vi "salRegSubEventsCMDsDL.vi"(8 "error in (no error)":errorcluster, 11 "MiddlewareSALThisComponent in":refnum<class "MiddlewareSALThisComponent.lvclass">) -> (0 "error out":errorcluster, 2 "Event Registration Refnum":refnum<event-registration>, 3 "MiddlewareSALThisComponent out":refnum<class "MiddlewareSALThisComponent.lvclass">)   [LabVIEW 2016, in "MiddlewareSALThisComponent.lvclass"]
uses:
  MiddlewareSALThisComponent.lvclass
  <vilib>/Utility/error.llb/DialogType.ctl
  ProgrammaticInitialization/ProgrammaticInitialization.lvclass
  ts_sallv_sedspectrometer/SALLV_calibrationSpectrometer.lvlib
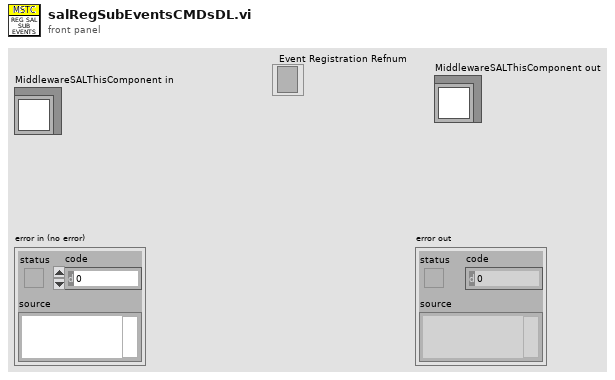
[diagram p1: front panel]
types:
  T1 = typedef "DialogType.ctl" = u16
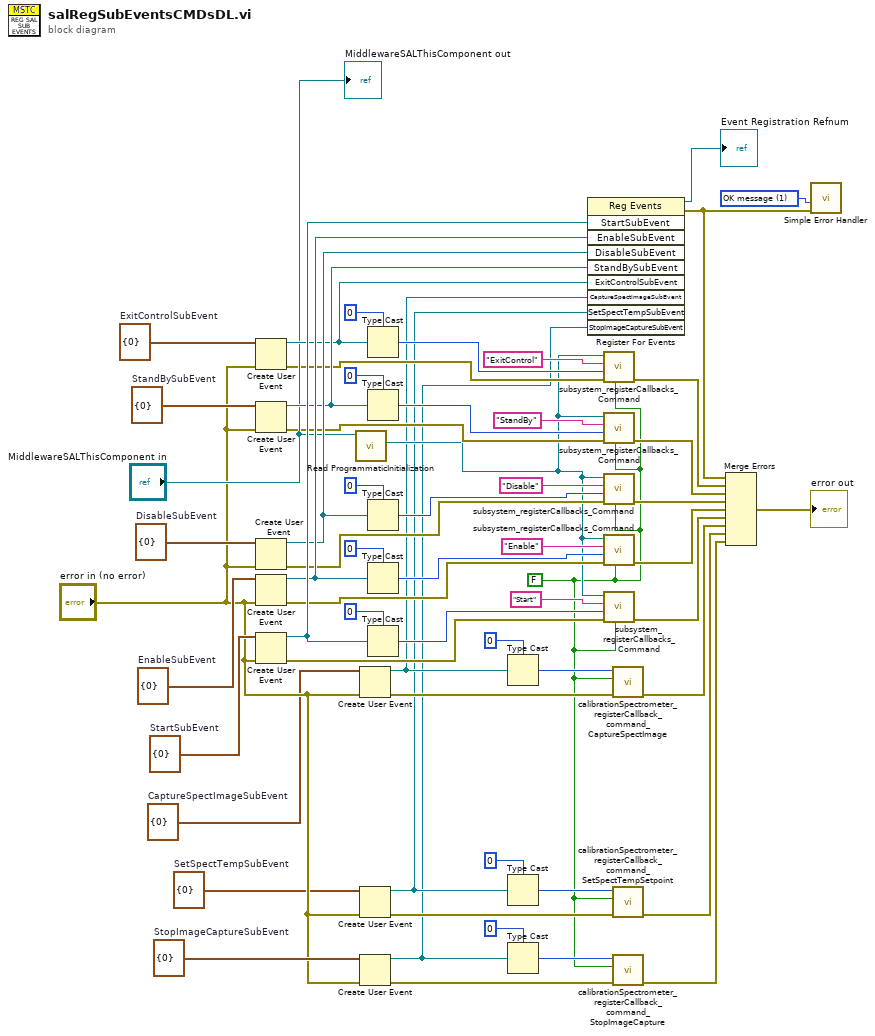
[diagram p0: block diagram]
diagram:
  w22 = cluster{"Data":i32} {"Data"=0}  # StopImageCaptureSubEvent
  w16 = cluster{"Data":i32} {"Data"=0}  # CaptureSpectImageSubEvent
  w20 = cluster{"Data":i32} {"Data"=0}  # SetSpectTempSubEvent
  w47 = cluster{"Data":i32} {"Data"=0}  # ExitControlSubEvent
  w49 = cluster{"Data":i32} {"Data"=0}  # StandBySubEvent
  w54 = cluster{"Data":i32} {"Data"=0}  # DisableSubEvent
  w57 = cluster{"Data":i32} {"Data"=0}  # EnableSubEvent
  w60 = cluster{"Data":i32} {"Data"=0}  # StartSubEvent
  w61 = T1 1 items=["no dialog", "OK message", "continue or stop message", "OK message + warnings", "continue/stop + warnings"] ("type of dialog (OK msg:1)")
  w4 = FALSE ("skipOld")
  n1 = Create User Event(user event datatype=w47, error in="error in (no error)") -> (user event=w46:refnum<user-event>, error out=w33:errorcluster)
  n2 = Create User Event(user event datatype=w49, error in="error in (no error)") -> (user event=w50:refnum<user-event>, error out=w32:errorcluster)
  n3 = Create User Event(user event datatype=w54, error in="error in (no error)") -> (user event=w52:refnum<user-event>, error out=w31:errorcluster)
  n4 = Create User Event(user event datatype=w57, error in="error in (no error)") -> (user event=w55:refnum<user-event>, error out=w28:errorcluster)
  n5 = Create User Event(user event datatype=w60, error in="error in (no error)") -> (user event=w58:refnum<user-event>, error out=w25:errorcluster)
  n6 = call-dynamic "Read ProgrammaticInitialization.vi"("MiddlewareSALThisComponent in"="MiddlewareSALThisComponent in") -> ("ProgrammaticInitialization"=w15:refnum<class "ProgrammaticInitialization.lvclass">)  [unwired: 8 in, 2 out]
  n7 = Create User Event(user event datatype=w16, error in="error in (no error)") -> (user event=w3:refnum<user-event>, error out=w12:errorcluster)
  n8 = Create User Event(user event datatype=w20, error in="error in (no error)") -> (user event=w2:refnum<user-event>, error out=w8:errorcluster)
  n9 = Create User Event(user event datatype=w22, error in="error in (no error)") -> (user event=w1:refnum<user-event>, error out=w7:errorcluster)
  n10 = Type Cast(type=0, x=w46) -> (*(type *) &x=w43:i32)
  n11 = Type Cast(type=0, x=w50) -> (*(type *) &x=w38:i32)
  n12 = Type Cast(type=0, x=w52) -> (*(type *) &x=w35:i32)
  n13 = Type Cast(type=0, x=w55) -> (*(type *) &x=w30:i32)
  n14 = Type Cast(type=0, x=w58) -> (*(type *) &x=w24:i32)
  n15 = Type Cast(type=0, x=w3) -> (*(type *) &x=w13:i32)
  n16 = Type Cast(type=0, x=w2) -> (*(type *) &x=w9:i32)
  n17 = Type Cast(type=0, x=w1) -> (*(type *) &x=w5:i32)
  n18 = register-events(w58, w55, w52, w50, w46, w3, w2, w1) -> (reference out=→"Event Registration Refnum":refnum<event-registration>, error out=w45:errorcluster)  [unwired: 2 in]
  n19 = call "subsystem_registerCallbacks_Command.vi"("skipOld"=w4, "error in (no error)"=w33, "handle"=w43, "topic"="ExitControl", "ProgrammaticInitialization in"=w15) -> ("error out"=w42:errorcluster)  [unwired: 5 in, 1 out]
  n20 = call "subsystem_registerCallbacks_Command.vi"("skipOld"=w4, "error in (no error)"=w32, "handle"=w38, "topic"="StandBy", "ProgrammaticInitialization in"=w15) -> ("error out"=w39:errorcluster)  [unwired: 5 in, 1 out]
  n21 = call "subsystem_registerCallbacks_Command.vi"("skipOld"=w4, "error in (no error)"=w31, "handle"=w35, "topic"="Disable", "ProgrammaticInitialization in"=w15) -> ("error out"=w36:errorcluster)  [unwired: 5 in, 1 out]
  n22 = call "subsystem_registerCallbacks_Command.vi"("skipOld"=w4, "error in (no error)"=w28, "handle"=w30, "topic"="Enable", "ProgrammaticInitialization in"=w15) -> ("error out"=w27:errorcluster)  [unwired: 5 in, 1 out]
  n23 = call "subsystem_registerCallbacks_Command.vi"("skipOld"=w4, "error in (no error)"=w25, "handle"=w24, "topic"="Start", "ProgrammaticInitialization in"=w15) -> ("error out"=w26:errorcluster)  [unwired: 5 in, 1 out]
  n24 = call "calibrationSpectrometer_registerCallback_command_CaptureSpectImage.vi"("error in (no error)"=w12, "skipOld"=w4, "handle"=w13) -> ("error out"=w11:errorcluster)  [unwired: 7 in, 1 out]
  n25 = call "calibrationSpectrometer_registerCallback_command_SetSpectTempSetpoint.vi"("error in (no error)"=w8, "skipOld"=w4, "handle"=w9) -> ("error out"=w10:errorcluster)  [unwired: 7 in, 1 out]
  n26 = call "calibrationSpectrometer_registerCallback_command_StopImageCapture.vi"("error in (no error)"=w7, "skipOld"=w4, "handle"=w5) -> ("error out"=w6:errorcluster)  [unwired: 7 in, 1 out]
  n27 = Merge Errors(w45, w42, w39, w36, w27, w26, w11, w10, w6) -> (→"error out":errorcluster)
  n28 = call <vilib>:"Simple Error Handler.vi"("type of dialog (OK msg:1)"=w61, "error in (no error)"=w45) -> ()  [unwired: 3 in, 5 out]
  "MiddlewareSALThisComponent out" <- "MiddlewareSALThisComponent in"
